vi "PathPlanner_FieldUtil_FieldSizeX.vi"() -> (3 "FieldSizeX_M":dbl)   [LabVIEW 2019, in "PathPlanner24.lvlib"]
doc: "The X size or length of the current field in meters\n\nInput:\n -- <none>\n\nOutputs:\n -- FieldSizeX -- X length of field (meters)"
uses:
  PathPlanner24.lvlib
  <vilib>/Rock Robotics/WPI/ThirdParty/JAS_Junk/TrajLib/Trajectory_Library.lvlib
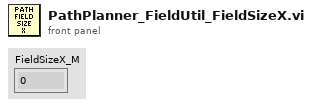
[diagram p1: front panel]
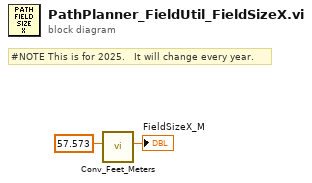
[diagram p0: block diagram]
diagram:
  # "#NOTE This is for 2025.   It will change every year."
  n1 = call <vilib>:"Conv_Feet_Meters.vi"("Feet"=57.573) -> ("Meters"=→"FieldSizeX_M":dbl)  [unwired: 10 in]
